vi "Read - Warning Input - Returns Same Warning.vi"() -> ()   [LabVIEW 2017, in "Generic Object Serializer Tests.lvlib" / "Serialization Binder.lvlib"]
uses:
  Serialization Binder.lvlib
  Generic Object Serializer/Generic Object Serializer.lvclass
  Generic Object Serializer/Read Serialization Binder.vi
  <vilib>/Utility/error.llb/Error Cluster From Error Code.vi
  <vilib>/ErrorRing/Error Ring.xnode
  Default Serialization Binder/Default Serialization Binder.lvclass
  Serialization Binder/Serialization Binder.lvclass
  <vilib>/addons/_JKI Toolkits/Caraya/classes/Test/Test.lvclass
  <vilib>/addons/_JKI Toolkits/Caraya/classes/Assert/Assert.lvclass
panel:
  out "error out":errorcluster
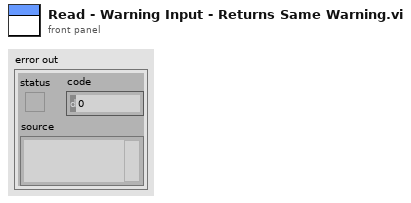
[diagram p1: front panel]
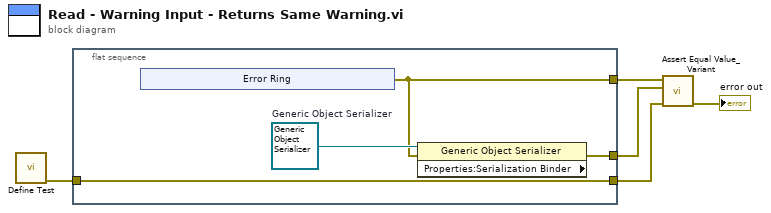
[diagram p0: block diagram]
diagram:
  n1 = call <vilib>:"Define Test.vi"() -> ("error out"=w4:errorcluster)  [unwired: 11 in]
  n2 = flat-sequence {
    tunnel: [w7] -> w5
    tunnel: w4 -> [w8]
    tunnel: [w8] -> w3
    tunnel: [w6] -> w1
    frame #0 {
      w9 = refnum<class "Generic Object Serializer.lvclass"> refnum  # Generic Object Serializer
      n3 = xnode "Error Ring"() -> ("error out"=w6:errorcluster)
      n4 = property class="Generic Object Serializer" props=["Properties:Serialization Binder"](reference=w9, error in=w6) -> (error out=w7:errorcluster)  [unwired: 2 out]
    }
  }
  n5 = call <vilib>:"Assert Equal Value_Variant.vi"("error in (no error)"=w3, "Y"=w5, "X"=w1) -> ("error out"=→"error out":errorcluster)  [unwired: 8 in]
